vi "tmds_Burst_Save_Test.vi"() -> ()   [LabVIEW 2020]
uses:
  <vilib>/Utility/TDMS File Viewer/NI_TDMS File Viewer.lvlib
panel:
  in  "Folder path":path
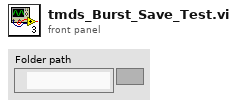
[diagram p1: front panel]
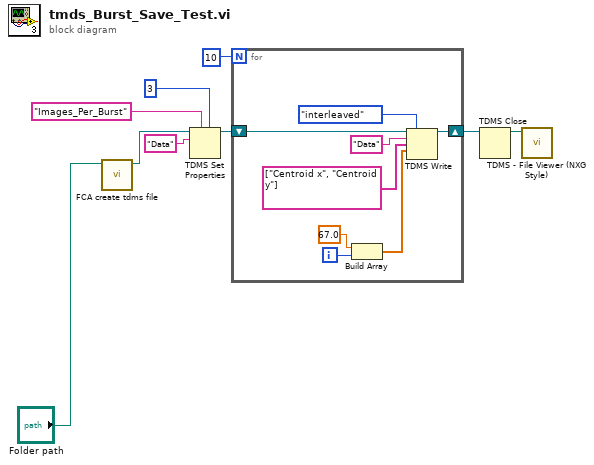
[diagram p0: block diagram]
diagram:
  n1 = call "FCA create tdms file.vi"("Folder path"="Folder path") -> ("Refnum out"=w9:refnum<k34>)  [unwired: 9 in, 1 out]
  n2 = TDMS Set Properties(5:3, 7:"Images_Per_Burst", 10:"Data" ("group name in (Untitled)"), 11:w9) -> (3:w7:refnum<k34>)  [unwired: 2 in, 3 out]
  n3 = for {
    N: 10 -> [_]
    shift-right: [w13] -> w5
    shift-left: w7 -> [w14]
    i -> [w10]
    n4 = Build Array(67.0 ("element"), w10) -> (w12:dbl[])
    n5 = TDMS Write(0:w14, 1:enum16{"decimated", "interleaved"}."interleaved" ("data layout (0:decimated)"), 5:"Data" ("group name in (Untitled)"), 7:string[] ["Centroid x", "Centroid y"] ("channel name(s) in (Untitled)"), 9:w12) -> (4:w13:refnum<k34>)  [unwired: 1 in, 3 out]
  }
  n6 = TDMS Close(11:w5) -> (3:w4:path)  [unwired: 1 in, 1 out]
  n7 = call <vilib>:"TDMS - File Viewer (NXG Style).vi"("file in"=w4) -> ()  [unwired: 9 in, 2 out]
